vi "TestTranslate.vi"() -> ()   [LabVIEW 2009]
uses:
  040 - SCREENS/00 - ButtonLibrary/BoutonModele.ctl
  Dictionnary/EnumCommandDictionnaire.ctl
panel:
  in  "Slide":dbl(slide) caption="Slide(T)" scale=0.0..10.0
  in  "Array":dbl[](array[numeric]) caption="Array(T)"
  in  "DictionnaryFile":path caption="DictionnaryFile(T)"
  out "error out":errorcluster caption="error out(T)"
  in  "Boolean 3":T1
  in  "Boolean 2":bool
  out "Array 2":cluster{"Boolean":bool}[](array[cluster]) caption="Array 2(T)"
  in  "Tab Control":enum32{"Page 1", "Page 2"}(tab) caption="Tab Control(T)"
  out "Test":T2 caption="Page 1(T)" {"Thermometer" scale=0.0..100.0}
  in  "Enum":enum16{""}(ring) caption="Enum(T)"
  in  "String":string caption="String(T)"
  in  "Boolean":bool caption="Boolean(T)"
  in  "Numeric":dbl caption="Numeric(T)"
  # "Coucou ..."
  # "Test ...(T)(T)(T)(T)(T)(T)(T)(T)(T)(T)(T)(T)(T)(T)(T)(T)(T)(T)(T)(T)(T)(T)(T)(T)(T)(T)(T)(T)(T)(T)(T)(T)(T)(T)(T)(T)(T)(T)(T)(T)(T)(T)(T)(T)(T)(T)(T)(T)(T)(T)(T)(T)(T)"
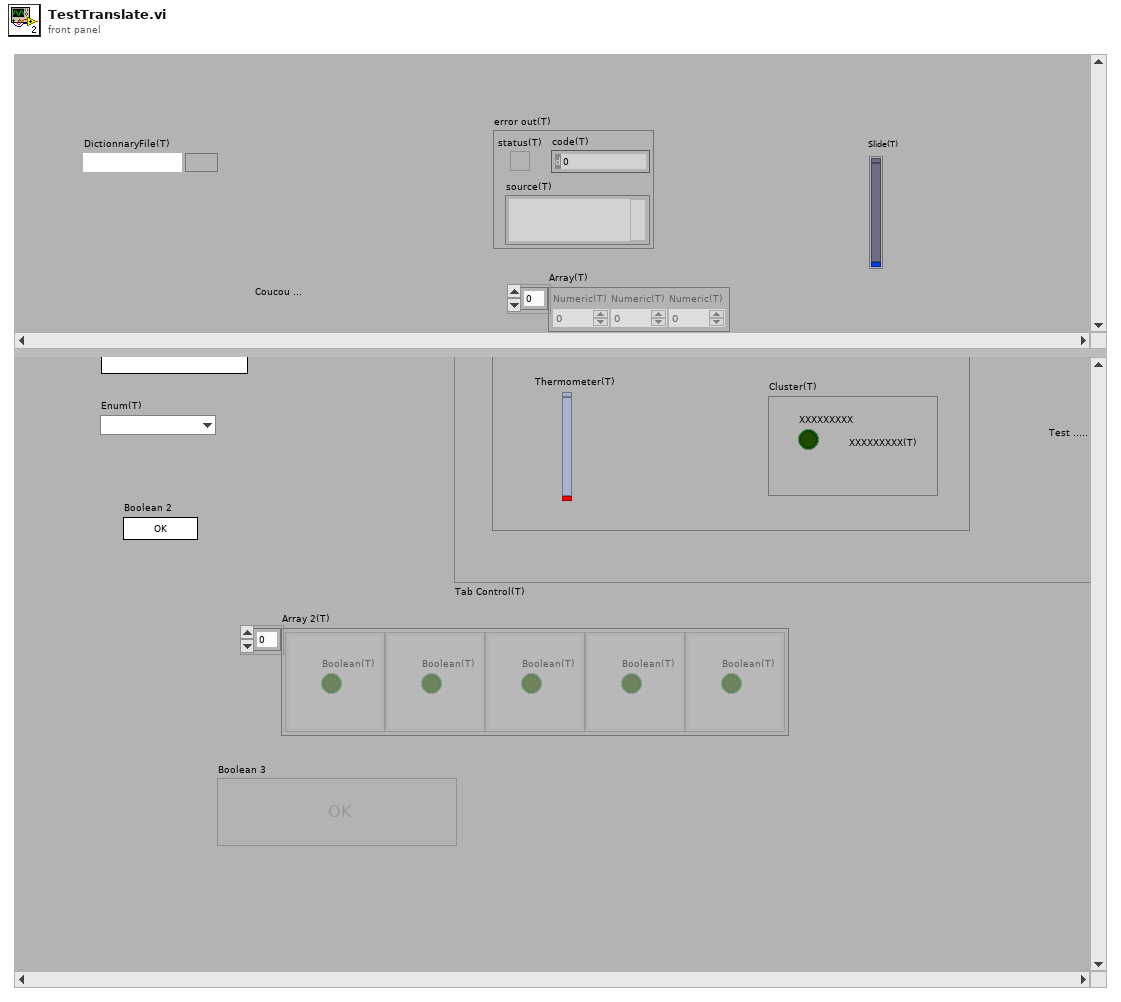
[diagram p1: front panel]
types:
  T1 = typedef "BoutonModele.ctl" = bool
  T2 = cluster{"Thermometer":dbl, "Cluster":cluster{"XXXXXXXXX":bool}}
  T3 = typedef "EnumCommandDictionnaire.ctl" = enum16{"Load", "Translate", "Save", "GetDico", "Set : A traduire = Vrai", "Set : A Traduire = Faux"}
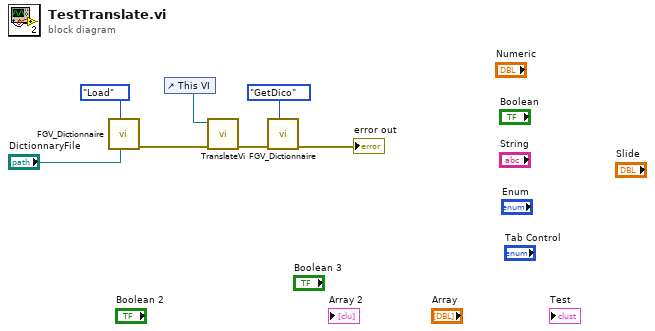
[diagram p0: block diagram]
diagram:
  n1 = call "FGV_Dictionnaire.vi"("FichierDictionnaire"="DictionnaryFile", "Command"=EnumCommandDictionnaire."Load") -> ("error out"=w7:errorcluster)  [unwired: 7 in, 2 out]
  n2 = control-ref of="This VI"() -> (w6:refnum<vi>)
  n3 = call "TranslateVi.vi"("error in (no error)"=w7, "VI ref"=w6) -> ("error out"=w3:errorcluster)  [unwired: 9 in]
  n4 = call "FGV_Dictionnaire.vi"("Command"=EnumCommandDictionnaire."GetDico", "error in (no error)"=w3) -> ("error out"=→"error out":errorcluster)  [unwired: 7 in, 2 out]
